vi "Example Output.vi"() -> ()   [LabVIEW 2010]
uses:
  C:/tf/play/labview/Tinkerforge.dll
panel:
  in  "uid":string="hf4"
  in  "port":i32=4223
  in  "host":string="localhost"
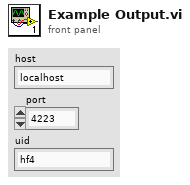
[diagram p1: front panel]
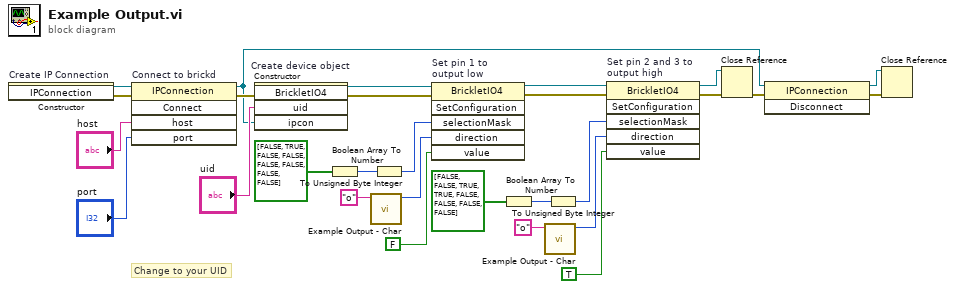
[diagram p0: block diagram]
diagram:
  # "Change to your UID"
  n1 = constructor on="Create IP Connection" class="IPConnection"() -> (reference out=w28:refnum<k24>, error out=w17:errorcluster)  [unwired: 3 in, 1 out]
  n2 = invoke on="Connect to brickd" class="IPConnection" method="Connect"(reference=w28, error in=w17, "host"="host", "port"="port") -> (reference out=w19:refnum<k24>, error out=w24:errorcluster)  [unwired: 1 in, 3 out]
  n3 = constructor on="Create device object" class="BrickletIO4"(error in=w24, "uid"="uid", "ipcon"=w19) -> (reference out=w22:refnum<k24>, error out=w23:errorcluster)  [unwired: 2 in, 3 out]
  n4 = Boolean Array To Number(Boolean array=bool[] [FALSE, TRUE, FALSE, FALSE, FALSE, FALSE, FALSE, FALSE]) -> (number=w15:u32)
  n5 = call "Example Output - Char.vi"("string"="o") -> ("char"=w5:u16)  [unwired: 10 in]
  n6 = To Unsigned Byte Integer(number=w15) -> (unsigned 8bit integer=w6:u8)
  n7 = invoke on="Set pin 1 to\noutput low" class="BrickletIO4" method="SetConfiguration"(reference=w22, error in=w23, "selectionMask"=w6, "direction"=w5, "value"=FALSE) -> (reference out=w12:refnum<k24>, error out=w13:errorcluster)  [unwired: 1 in, 4 out]
  n8 = Boolean Array To Number(Boolean array=bool[] [FALSE, FALSE, TRUE, TRUE, FALSE, FALSE, FALSE, FALSE]) -> (number=w7:u32)
  n9 = call "Example Output - Char.vi"("string"="o") -> ("char"=w2:u16)  [unwired: 10 in]
  n10 = To Unsigned Byte Integer(number=w7) -> (unsigned 8bit integer=w3:u8)
  n11 = invoke on="Set pin 2 and 3 to\noutput high" class="BrickletIO4" method="SetConfiguration"(reference=w12, error in=w13, "selectionMask"=w3, "direction"=w2, "value"=TRUE) -> (reference out=w11:refnum<k24>, error out=w10:errorcluster)  [unwired: 1 in, 4 out]
  n12 = Close Reference(reference=w11, error in (no error)=w10) -> (error out=w21:errorcluster)
  n13 = invoke class="IPConnection" method="Disconnect"(reference=w19, error in=w21) -> (reference out=w18:refnum<k24>, error out=w20:errorcluster)  [unwired: 1 in, 1 out]
  n14 = Close Reference(reference=w18, error in (no error)=w20) -> ()  [unwired: 1 out]
